vi "getDeviceName.vi"(8 "error in (no error)":errorcluster, 11 "reference (in)":refnum<class "_Controller.lvclass">) -> (0 "error out":errorcluster, 2 "deviceName":string, 3 "reference (out)":refnum<class "_Controller.lvclass">)   [LabVIEW 2020, in "classes.lvlib" / "_Controller.lvclass"]
doc: "Produced By:\n\n<B>Kod Integrations, LLC</B>\n4835 Marianne Drive\nMount Airy, MD 21771\nhttp://www.kodintegrations.com\nemail: info@kodintegrations.com\nphone: (240) 687-1288"
uses:
  _Controller.lvclass
  _Controller.lvclass/_Controller.ctl
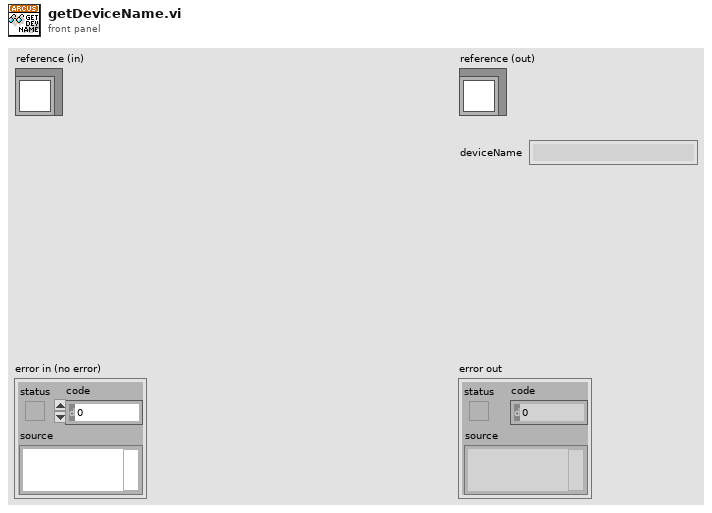
[diagram p1: front panel]
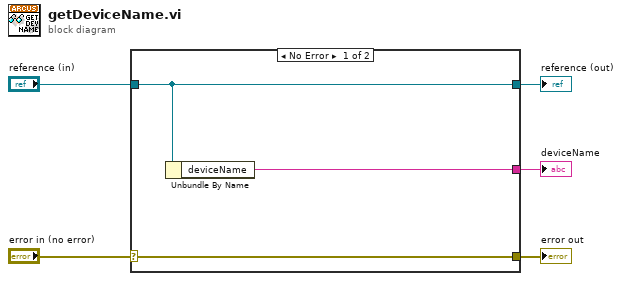
[diagram p0: block diagram]
diagram:
  n1 = case shown="No Error" "error in (no error)" {
    selector: "error in (no error)" -> [w8 w9]
    tunnel: [w8 w9] -> w4
    tunnel: [w7 w10] -> w2
    tunnel: "reference (in)" -> [w7 w10]
    tunnel: [w6 _] -> w1
    frame No Error {
      n2 = Unbundle By Name(w7) -> ("deviceName"=w6:string)
    }
    frame Error {
    }
  }
  "error out" <- w4
  "reference (out)" <- w2
  "deviceName" <- w1
